vi "dequeueMessage.vi"(8 "error in (no error)":errorcluster) -> (0 "error out":errorcluster, 3 "Message out":T1)   [LabVIEW 2017, in "lowLevelController.lvlib"]
uses:
  lowLevelController.lvlib
  TypeDefs/message.ctl
  TypeDefs/queueFGVState.ctl
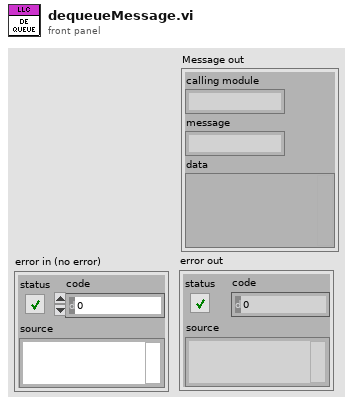
[diagram p1: front panel]
types:
  T1 = typedef "lowLevelController.lvlib/message.ctl" = cluster{"calling module":string, "message":string, "data":variant}
  T2 = typedef "lowLevelController.lvlib/queueFGVState.ctl" = enum16{"set", "get"}
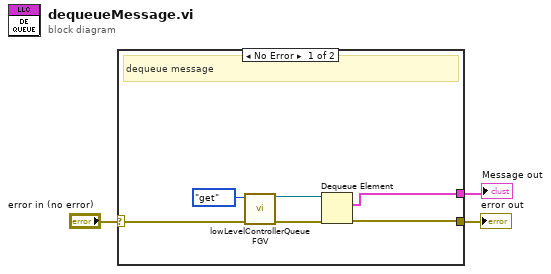
[diagram p0: block diagram]
diagram:
  n1 = case shown="No Error" "error in (no error)" {
    selector: "error in (no error)" -> [w9 w10]
    tunnel: [w7 w10] -> w2
    tunnel: [w5 _] -> w1
    frame No Error {
      # "dequeue message"
      n2 = call "lowLevelControllerQueueFGV.vi"("error in (no error)"=w9, 11:queueFGVState."get") -> ("error out"=w8:errorcluster, "queue out"=w6:refnum<queue>)  [unwired: 8 in]
      n3 = Dequeue Element(queue=w6, error in (no error)=w8) -> (element=w5:T1, error out=w7:errorcluster)  [unwired: 1 in, 2 out]
    }
    frame Error {
    }
  }
  "error out" <- w2
  "Message out" <- w1
